vi "save stats to INI (SubVI).vi"(7 "lastSamp":i32, 8 "errIN":errorcluster, 10 "lastShot":i32, 11 "configPath":path) -> (0 "errOUT":errorcluster, 3 "recordNum":dbl)   [LabVIEW 2015]
uses:
  <vilib>/Utility/config.llb/Write Key (I32).vi
  <vilib>/Utility/config.llb/NI_LVConfig.lvlib
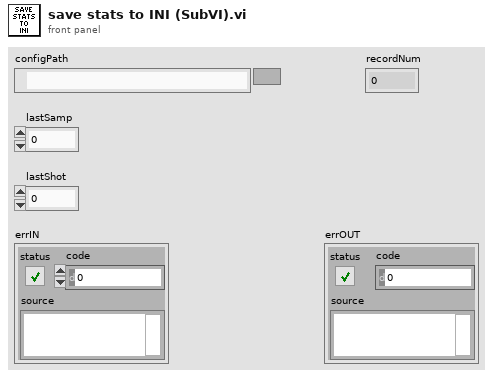
[diagram p1: front panel]
types:
  T1 = typedef "NI_LVConfig.lvlib/Config Data RefNum.ctl" = refnum<k1>
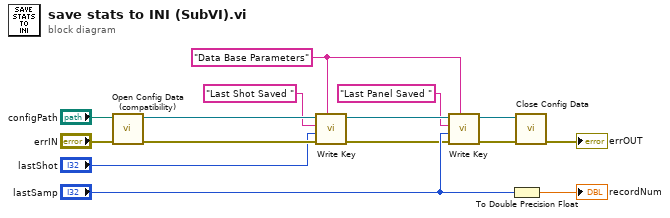
[diagram p0: block diagram]
diagram:
  w9 = "Data Base Parameters" ("section")
  n1 = call <vilib>:"Open Config Data (compatibility).vi"("error in (no error)"="errIN", "configuration file path"="configPath") -> ("error out"=w5:errorcluster, "refnum"=w6:T1)  [unwired: 7 in, 1 out]
  n2 = call-poly <vilib>:"Write Key.vi"("section"=w9, "error in (no error)"=w5, "value"="lastShot", "key"="Last Shot Saved ", "refnum"=w6) -> ("error out"=w7:errorcluster, "refnum out"=w8:T1)  [unwired: 5 out]
  n3 = call-poly <vilib>:"Write Key.vi"("section"=w9, "error in (no error)"=w7, "value"="lastSamp", "key"="Last Panel Saved ", "refnum"=w8) -> ("error out"=w14:errorcluster, "refnum out"=w1:T1)  [unwired: 5 out]
  n4 = To Double Precision Float(number="lastSamp") -> (double precision float=→"recordNum":dbl)
  n5 = call <vilib>:"Close Config Data.vi"("error in (no error)"=w14, "refnum"=w1) -> ("error out"=→"errOUT":errorcluster)  [unwired: 1 in, 8 out]
